vi "MainV1.vi"() -> ()   [LabVIEW 2016]
uses:
  Control/StreamCluster.ctl
  Control/GUICluster.ctl
  Control/Fahrart.ctl
  <vilib>/dex/Stream Element Allocation Mode.ctl
  <vilib>/myRIO/Instrument Drivers/Onboard IO/AI/typedefs/AI Reference.ctl
  <vilib>/myRIO/Common/Instrument Driver Framework/Utilities/typedefs/myRIO Generic Hardware Reference.ctl
  <vilib>/myRIO/Common/Instrument Driver Framework/Utilities/typedefs/Hardware Version Enum.ctl
  <vilib>/myRIO/Common/Instrument Driver Framework/Utilities/typedefs/myRIO v1.0 Reference.ctl
  <vilib>/myRIO/Common/Instrument Driver Framework/Utilities/typedefs/Generic FPGA Reference.ctl
  <vilib>/myRIO/Common/Instrument Driver Framework/myRIO v1.0/AI/typedefs/AI Channels List.ctl
  <vilib>/myRIO/Common/Instrument Driver Framework/myRIO v1.0/AI/typedefs/AI Channels Enum.ctl
  <vilib>/myRIO/Common/Instrument Driver Framework/Utilities/typedefs/Analog Scaling Constants List.ctl
  <vilib>/myRIO/Common/Instrument Driver Framework/Utilities/typedefs/Analog Scaling Constants.ctl
  <vilib>/userdefined/High Color/nirio_resource_hc.ctl
  <vilib>/myRIO/Instrument Drivers/Onboard IO/PWM/typedefs/PWM Reference.ctl
  <vilib>/myRIO/Common/Instrument Driver Framework/myRIO v1.0/PWM/typedefs/PWM Channels Enum.ctl
  <vilib>/myRIO/Instrument Drivers/Onboard IO/PWM/typedefs/PWM Configuration.ctl
  <vilib>/myRIO/Common/Instrument Driver Framework/Utilities/vis/Is FPGA Ref Available.vi
  <vilib>/myRIO/Common/Instrument Driver Framework/myRIO v1.0/AI/vis/myRIO v1.1 Open AI.vi
  <vilib>/myRIO/Instrument Drivers/Onboard IO/AI/vis/Read.vi
  <vilib>/myRIO/Common/Instrument Driver Framework/myRIO v1.0/PWM/vis/myRIO v1.1 Open PWM.vi
  <vilib>/myRIO/Instrument Drivers/Onboard IO/PWM/vis/Set Duty Cycle and Frequency.vi
  <vilib>/myRIO/Common/Instrument Driver Framework/Utilities/vis/Validate Channels.vi
  <vilib>/myRIO/Common/Instrument Driver Framework/myRIO v1.0/AI/vis/myRIO v1.0 Reserve AI.vi
  <vilib>/myRIO/Common/Instrument Driver Framework/myRIO v1.0/PWM/vis/myRIO v1.0 Reserve PWM.vi
  <vilib>/myRIO/Common/Instrument Driver Framework/myRIO v1.0/AI/vis/myRIO v1.0 Build MUX Configuration AI.vi
  <vilib>/myRIO/Common/Instrument Driver Framework/myRIO v1.0/Resource Manager/vis/myRIO v1.0 Reserve Channel List.vi
  <vilib>/myRIO/Common/Instrument Driver Framework/myRIO v1.0/PWM/vis/myRIO v1.0 Build MUX Configuration PWM.vi
  <vilib>/myRIO/Common/Instrument Driver Framework/myRIO v1.0/Resource Manager/vis/myRIO v1.0 Reserve Channel.vi
  <vilib>/myRIO/Common/Instrument Driver Framework/myRIO v1.0/Resource Manager/vis/myRIO v1.0 Unreserve Channel.vi
  <vilib>/myRIO/Common/Instrument Driver Framework/myRIO v1.0/Resource Manager/vis/myRIO v1.0 Create Configuration List.vi
  <vilib>/myRIO/Common/Instrument Driver Framework/myRIO v1.0/Resource Manager/vis/myRIO v1.0 Build Mutex Name.vi
  <vilib>/Utility/VariantDataType/GetNumericInfo.vi
  <vilib>/Utility/error.llb/Error Cluster From Error Code.vi
  <vilib>/myRIO/Common/Instrument Driver Framework/myRIO v1.0/myRIO v1.1 Open.vi
  <vilib>/myRIO/Common/Instrument Driver Framework/Utilities/vis/IO Manager.vi
  <vilib>/myRIO/Common/Instrument Driver Framework/Utilities/vis/Configuration Manager.vi
  <vilib>/myRIO/Common/Instrument Driver Framework/myRIO v1.0/Resource Manager/vis/myRIO v1.0 Configure IO.vi
  <vilib>/myRIO/Common/Instrument Driver Framework/myRIO v1.0/myRIO v1.0 Close.vi
  <vilib>/myRIO/Common/Instrument Driver Framework/myRIO v1.0/PWM/vis/myRIO v1.0 Write PWM.vi
  <vilib>/myRIO/Common/Instrument Driver Framework/myRIO v1.0/AI/vis/myRIO v1.0 Get Scaling Constants AI.vi
  <vilib>/myRIO/Common/Instrument Driver Framework/myRIO v1.0/AI/vis/myRIO v1.0 Read AI.vi
  <vilib>/myRIO/Express VI/Onboard IO/PWM/PWM Express VI.xnode
  <vilib>/myRIO/Instrument Drivers/Onboard IO/PWM/vis/myRIO PWM Open.xnode
  <vilib>/myRIO/Express VI/Onboard IO/AI/AI Express VI.xnode
  <vilib>/myRIO/Instrument Drivers/Onboard IO/AI/vis/myRIO AI Open.xnode
  <vilib>/myRIO/Instrument Drivers/Onboard IO/PWM/PWM.lvlib
  <vilib>/myRIO/Instrument Drivers/Onboard IO/AI/AI.lvlib
panel:
  out "GUIInput":T1={"Fahrart"=enum."Überholen", "Geschwindigkeitsmultiplikator"=0.0, "Stop"=TRUE, "Automatisch"=FALSE}
  out "output":T3
  out "Drehzahl":dbl(knob) scale=0.0..15000.0
  out "Stop":bool
  out "Impulse pro Minute":dbl
  out "counter":dbl=1170.0
  out "Leistung":dbl=6.577122973792136
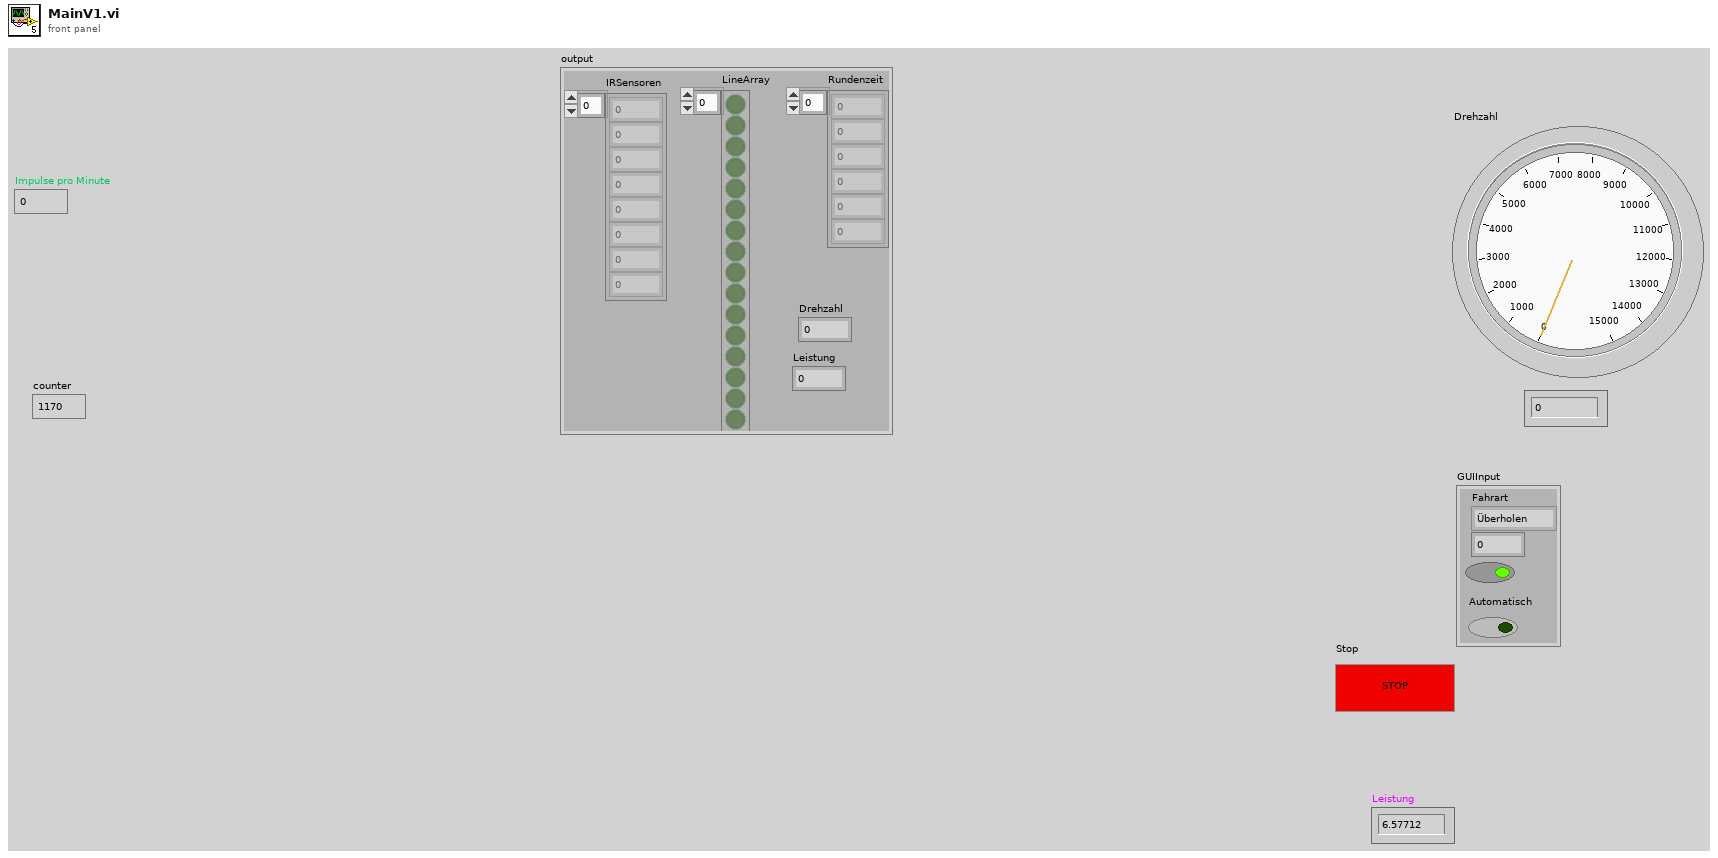
[diagram p1: front panel]
types:
  T1 = typedef "GUICluster.ctl" = cluster{"Fahrart":T2, "Geschwindigkeitsmultiplikator":dbl, "Stop":bool, "Automatisch":bool}
  T2 = typedef "Fahrart.ctl" = enum16{"Fahren Array", "Folgen", "Überholen"}
  T3 = typedef "StreamCluster.ctl" = cluster{"IRSensoren":dbl[], "LineArray":bool[], "Rundenzeit":dbl[], "Drehzahl":dbl, "Leistung":dbl}
  T4 = typedef "Stream Element Allocation Mode.ctl" = u32
  T5 = typedef "PWM.lvlib/PWM Reference.ctl" = cluster{"myRIO Reference":T6, "PWM Channels Enum":T10, "PWM Configuration":T11}
  T6 = typedef "myRIO Generic Hardware Reference.ctl" = cluster{"myRIO Model":T7, "myRIO Hardware Reference":T8}
  T7 = typedef "Hardware Version Enum.ctl" = enum16{"Unknown", "myRIO-1900", "myRIO-1950", "roboRIO", "NI ELVIS RIO CM"}
  T8 = typedef "myRIO v1.0 Reference.ctl" = cluster{"Generic FPGA Reference":T9, "Allow multiple opens":bool}
  T9 = typedef "Generic FPGA Reference.ctl" = refnum<k20>
  T10 = typedef "PWM Channels Enum.ctl" = enum16{"Not Connected", "C/PWM0", "C/PWM1", "A/PWM0", "A/PWM1", "A/PWM2", "B/PWM0", "B/PWM1", "B/PWM2", "PWM/PWM0", "PWM/PWM1", "PWM/PWM2", "PWM/PWM3", "PWM/PWM4", "PWM/PWM5", "PWM/PWM6", "PWM/PWM7", "PWM/PWM8", "PWM/PWM9"}
  T11 = typedef "PWM.lvlib/PWM Configuration.ctl" = cluster{"Frequency":dbl, "Duty Cycle":dbl}
  T12 = typedef "nirio_resource_hc.ctl" = tag
  T13 = typedef "AI.lvlib/AI Reference.ctl" = cluster{"myRIO Reference":T6, "AI Channels List":T14, "AI Scaling Constants List":T16}
  T14 = typedef "AI Channels List.ctl" = T15[]
  T15 = typedef "AI Channels Enum.ctl" = enum16{"Not Connected", "AudioIn/Left", "AudioIn/Right", "C/AI0", "C/AI1", "A/AI0", "A/AI1", "A/AI2", "A/AI3", "B/AI0", "B/AI1", "B/AI2", "B/AI3", "AI/AI0", "AI/AI1", "AI/AI2", "AI/AI3"}
  T16 = typedef "Analog Scaling Constants List.ctl" = T17[]
  T17 = typedef "Analog Scaling Constants.ctl" = cluster{"LSB Weight (Volts)":dbl, "Offset (Volts)":dbl, "Signed?":bool}
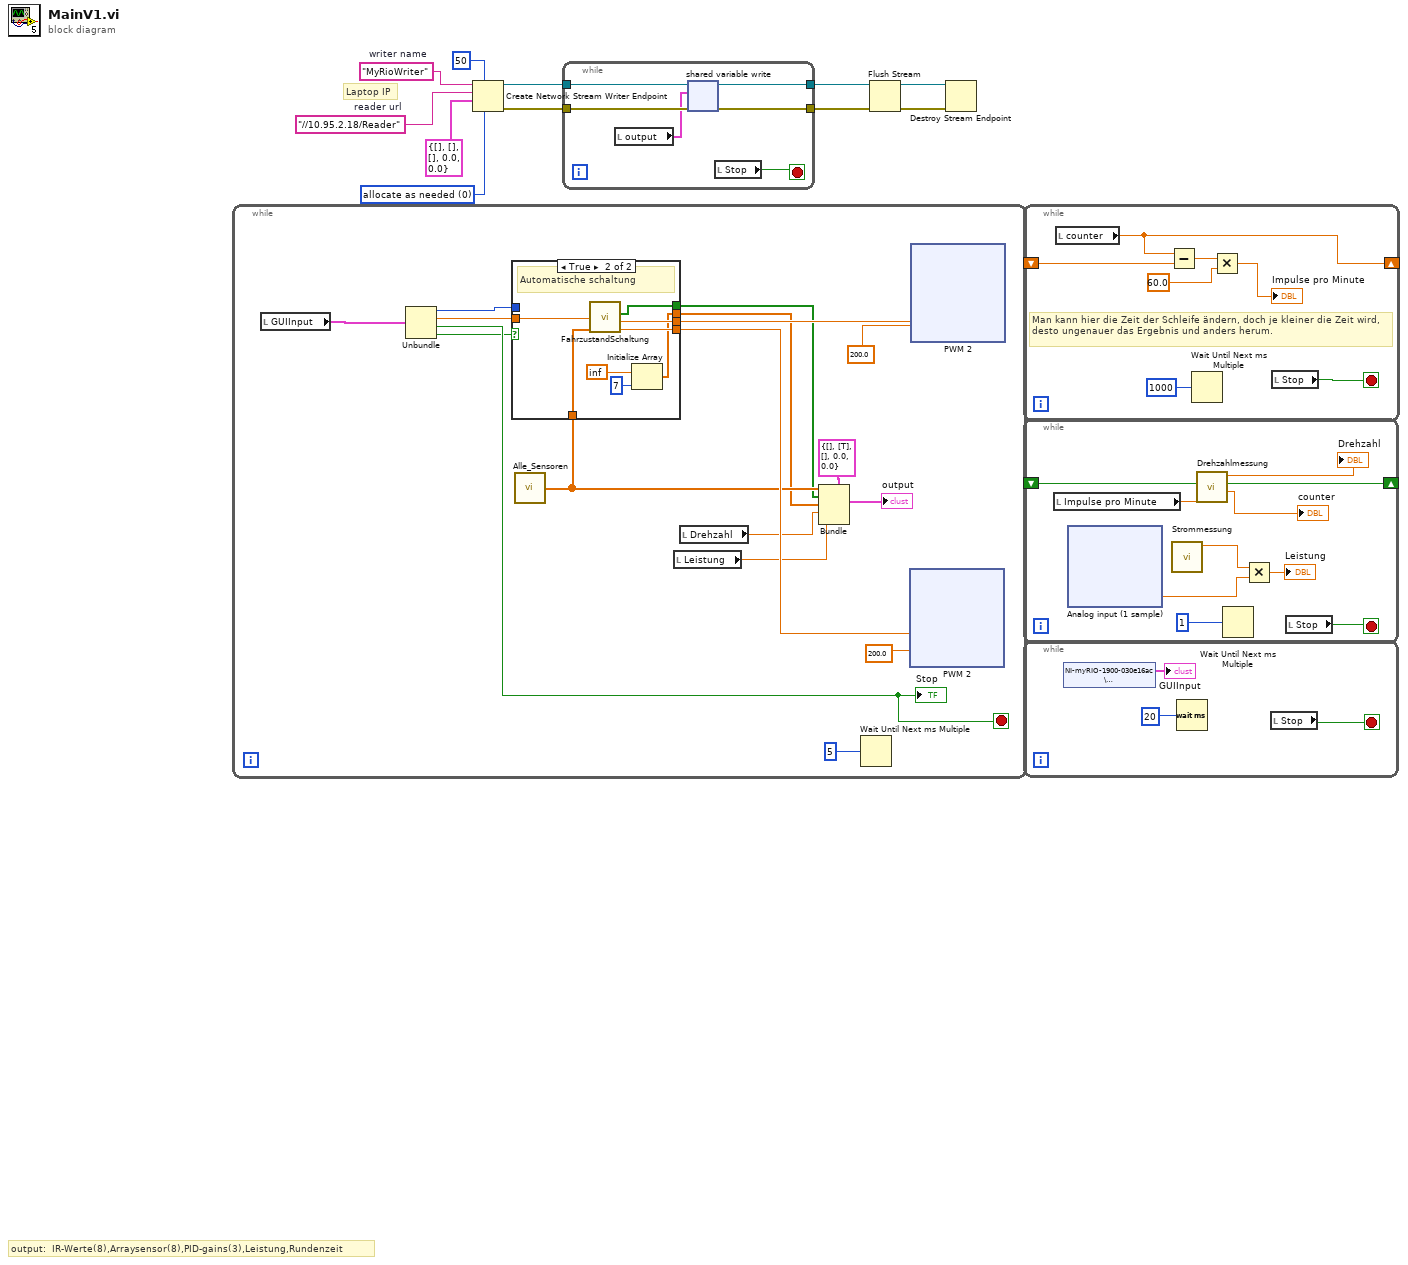
[diagram p0: block diagram]
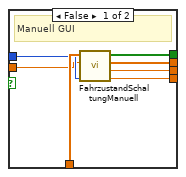
[diagram p2: hidden frame]
diagram:
  w7 = T4 0 items=["allocate as needed", "pre-allocate"] ("element allocation mode")
  w10 = "//10.95.2.18/Reader"  # reader url
  w11 = "MyRioWriter"  # writer name
  # "Laptop IP"
  # "output:  IR-Werte(8),Arraysensor(8),PID-gains(3),Leistung,Rundenzeit"
  n1 = while {
    stop <- w22 stop-if-true
    n2 = local read "GUIInput"() -> (w13:T1)
    n3 = Unbundle(w13) -> ("Fahrart"=w23:T2, "Geschwindigkeitsmultiplikator"=w15:dbl, "Stop"=w22:bool, "Automatisch"=w12:bool)
    "Stop" <- w22
    n4 = call "Alle_Sensoren.vi"() -> ("Array"=w19:dbl[])  [unwired: 5 in]
    n5 = case shown="True" w12 {
      tunnel: w23 -> [w34 _]
      tunnel: [w31 w43] -> w25
      tunnel: w19 -> [w35 w42]
      tunnel: [w33 w39] -> w18
      tunnel: [w32 w36] -> w14
      tunnel: [w30 w41] -> w24
      tunnel: w15 -> [w29 w40]
      frame False {
        # "Manuell GUI"
        n6 = call "FahrzustandSchaltungManuell.vi"("Fahrzustand"=w34, "Geschwindigkeitsmultiplikator"=w29, "Sensoren"=w35) -> ("PWM Motor"=w30:dbl, "PWM Lenkung"=w31:dbl, "Rundenzeiten"=w32:dbl[], "Linefollow_Array"=w33:bool[])  [unwired: 5 in]
      }
      frame True {
        # "Automatische schaltung"
        n7 = call "FahrzustandSchaltung.vi"("Sensoren"=w42, "Geschwindigkeitsmultiplikator"=w40) -> ("PWM Motor"=w41:dbl, "PWM Lenkung"=w43:dbl, "Linefollow_Array"=w39:bool[])  [unwired: 3 in]
        n8 = Initialize Array(inf, 7 ("dimension size")) -> (w36:dbl[])
      }
    }
    n9 = local read "Leistung"() -> (w16:dbl)
    n10 = local read "Drehzahl"() -> (w17:dbl)
    n11 = Bundle(cluster=T3 {"IRSensoren"=[], "LineArray"=[TRUE], "Rundenzeit"=[], "Drehzahl"=0.0, "Leistung"=0.0} ("Cluster"), "IRSensoren"=w19, "LineArray"=w18, "Rundenzeit"=w14, "Drehzahl"=w17, "Leistung"=w16) -> (→"output":T3)
    n12 = Wait Until Next ms Multiple(millisecond multiple=u32 5) -> ()  [unwired: 1 out]
    n13 = xnode "PWM 2"("Duty Cycle"=w24, "Frequency [Hz]"=200.0) -> ()  [unwired: 1 in, 1 out]
    n14 = xnode "PWM 2"("Duty Cycle"=w25, "Frequency [Hz]"=200.0 ("y")) -> ()  [unwired: 1 in, 1 out]
  }
  n15 = Create Network Stream Writer Endpoint(6:w7, 7:50 ("writer buffer size"), 9:T3 {"IRSensoren"=[], "LineArray"=[], "Rundenzeit"=[], "Drehzahl"=0.0, "Leistung"=0.0} ("Cluster"), 10:w10, 11:w11) -> (0:w3:errorcluster, 3:w4:refnum<k21>)  [unwired: 2 in]
  n16 = while {
    tunnel: w4 -> [w119]
    tunnel: w3 -> [w118]
    tunnel: [w117] -> w2
    tunnel: [w116] -> w1
    stop <- w114 stop-if-true
    n17 = local read "output"() -> (w115:T3)
    n18 = shared-variable-write(w119, w118, w115) -> (w117:refnum<k21>, w116:errorcluster)  [unwired: 1 in, 1 out]
    n19 = local read "Stop"() -> (w114:bool)
  }
  n20 = Flush Stream(8:w1, 11:w2) -> (0:w6:errorcluster, 3:w5:refnum<k21>)  [unwired: 2 in, 1 out]
  n21 = Destroy Stream Endpoint(8:w6, 11:w5) -> ()  [unwired: 1 out]
  n22 = while {
    shift-right: [w125] -> _
    shift-left: _ -> [w124]
    stop <- w121 stop-if-true
    # "Man kann hier die Zeit der Schleife ändern, doch je kleiner die Zeit wird, desto ungenauer das Ergebnis und anders herum."
    n23 = local read "counter"() -> (w125:dbl)
    n24 = Subtract(x=w125, y=w124) -> (x-y=w122:dbl)
    n25 = Wait Until Next ms Multiple(millisecond multiple=u32 1000 ("Vielfache von ms")) -> ()  [unwired: 1 out]
    n26 = Multiply(x=w122, y=60.0) -> (x*y=→"Impulse pro Minute":dbl)
    n27 = local read "Stop"() -> (w121:bool)
  }
  n28 = while {
    shift-right: [w129] -> _
    shift-left: _ -> [w128]
    stop <- w130 stop-if-true
    n29 = local read "Impulse pro Minute"() -> (w135:dbl)
    n30 = xnode "Analog input (1 sample)"() -> ("C/AI0 (AI0)"=w133:dbl)  [unwired: 1 in, 1 out]
    n31 = call "Strommessung.vi"() -> ("Strom"=w131:dbl)  [unwired: 10 in, 1 out]
    n32 = call "Drehzahlmessung.vi"("Impuls per Minute"=w135, "in"=w128) -> ("counter"=→"counter":dbl, "out"=w129:bool, "Drehzahl"=→"Drehzahl":dbl)  [unwired: 6 in]
    n33 = Wait Until Next ms Multiple(millisecond multiple=u32 1 ("milliseconds to wait")) -> ()  [unwired: 1 out]
    n34 = Multiply(x=w131, y=w133) -> (x*y=→"Leistung":dbl)
    n35 = local read "Stop"() -> (w130:bool)
  }
  n36 = while {
    stop <- w176 stop-if-true
    n37 = shared-variable "NI-myRIO-1900-030e16ac\\GUICommunicationLibrary.lvlib\\GUIInput"() -> (→"GUIInput":T1)  [unwired: 1 in, 1 out]
    n38 = Wait (ms)(milliseconds to wait=u32 20) -> ()  [unwired: 1 out]
    n39 = local read "Stop"() -> (w176:bool)
  }
